vi "load.jsons.vi"() -> ()   [LabVIEW 2024]
uses:
  definitions/seriesJSON.ctl
  definitions/seriesInfo.ctl
  definitions/issueInfo.ctl
  definitions/creator.ctl
  definitions/character.ctl
  definitions/team.ctl
  definitions/location.ctl
  definitions/concept.ctl
  definitions/thing.ctl
  definitions/storyArc.ctl
  <vilib>/addons/_JKI.lib/Serialization/JSON/JKI JSON Serialization.lvlib
  series_class/series_class.lvclass
panel:
  out "error out":errorcluster
  out "event map out":map{string, set{string}}(c390)
  out "current series":string
  out "char map out":map{string, set{string}}(c390)
  in  "Path":path=path "D:/Comics/data/comicvine"
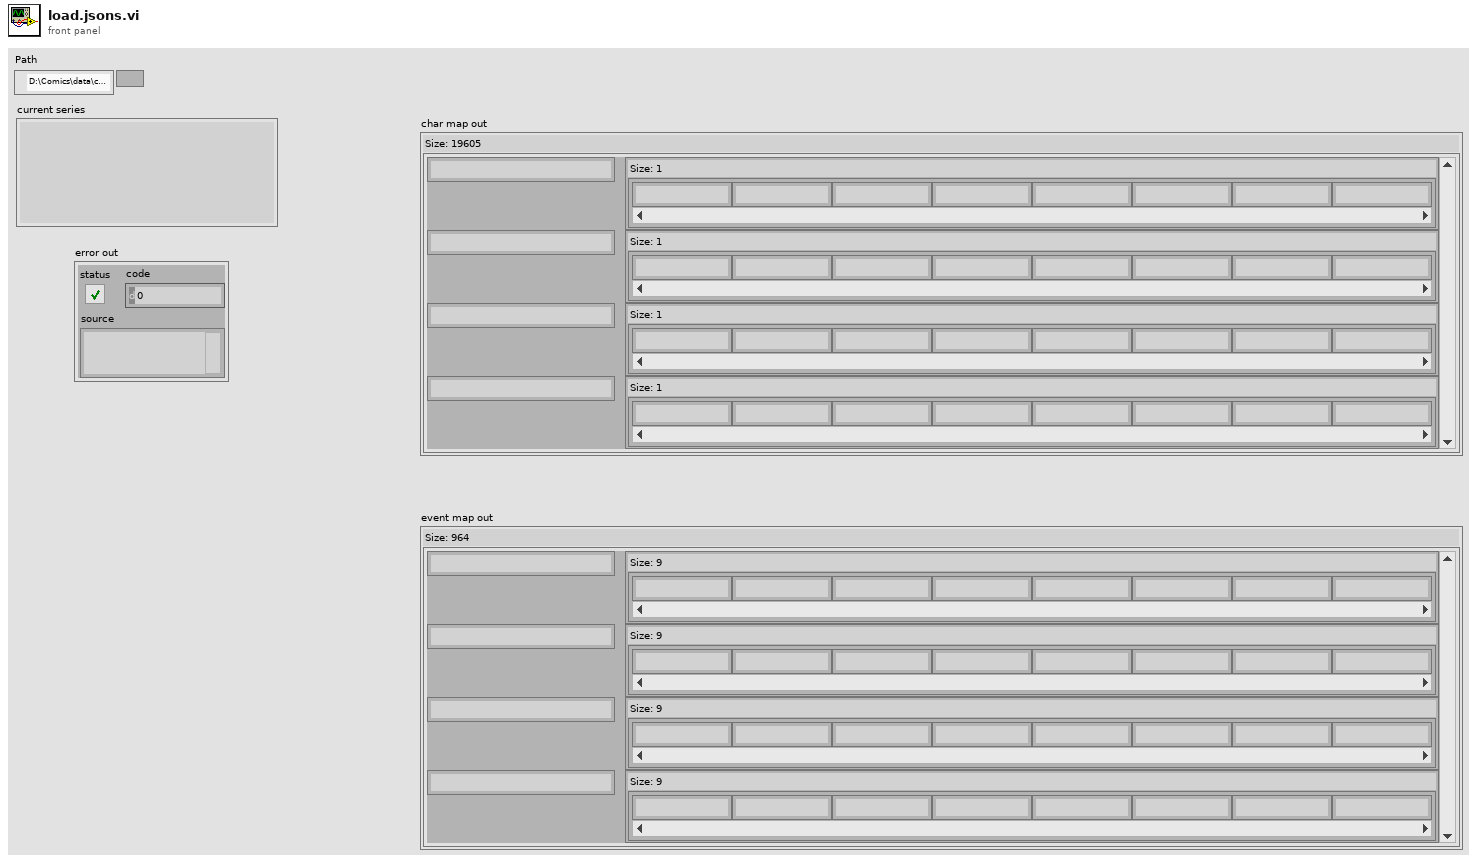
[diagram p1: front panel]
types:
  T1 = enum16{"open", "replace", "create", "open or create", "replace or create", "replace or create with confirmation"}
  T2 = cluster{"characters":cluster{"character":string, "issueIDs":string[]}[], "storyArcs":cluster{"storyArc":string, "issueIDs":string[]}[]}
  T3 = typedef "seriesJSON.ctl" = cluster{"seriesInfo":T4, "issueInfo":T5[]}
  T4 = typedef "seriesInfo.ctl" = cluster{"title":string, "base url":string, "publisher":string, "publisher url":string, "count":i32, "start year":i32, "volume":i32}
  T5 = typedef "issueInfo.ctl" = cluster{"cover date":timestamp, "release date":timestamp, "number":string, "url":string, "small cover url":string, "name":string, "large cover url":string, "id":string, "creators":T6[], "characters":T7[], "teams":T8[], "locations":T9[], "concepts":T10[], "objects":T11[], "storyArcs":T12[], "description":string}
  T6 = typedef "creator.ctl" = cluster{"name":string, "role":string, "url":string}
  T7 = typedef "character.ctl" = cluster{"name":string, "url":string}
  T8 = typedef "team.ctl" = cluster{"name":string, "url":string}
  T9 = typedef "location.ctl" = cluster{"name":string, "url":string}
  T10 = typedef "concept.ctl" = cluster{"name":string, "url":string}
  T11 = typedef "thing.ctl" = cluster{"name":string, "url":string}
  T12 = typedef "storyArc.ctl" = cluster{"name":string, "url":string}
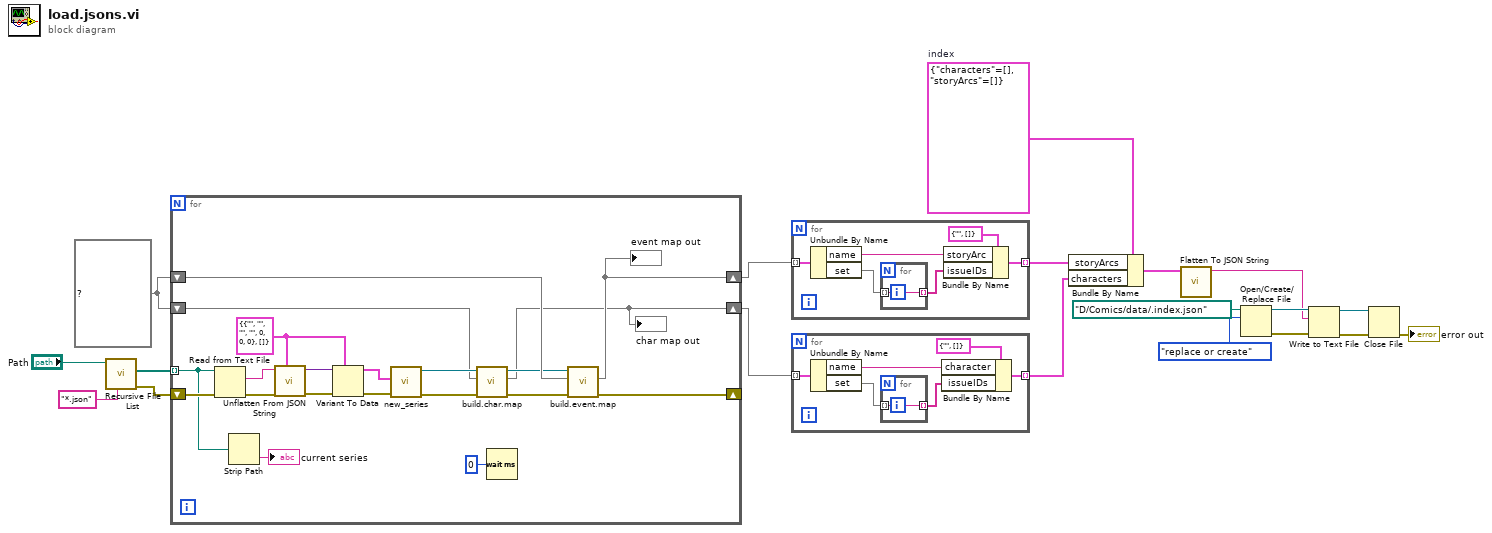
[diagram p0: block diagram]
diagram:
  w12 = T2 {"characters"=[], "storyArcs"=[]}  # index
  w15 = map{string, set{string}} {} ("char map in")
  n1 = call <vilib>:"Recursive File List.vi"("pattern"="*.json", "Folder Path"="Path") -> ("error out"=w16:errorcluster, "All Files in Dir"=w17:path[])  [unwired: 5 in, 3 out]
  n2 = for {
    tunnel: w17 -> [w28] mode=indexing
    shift-right: [w24] -> _
    shift-left: w16 -> [w39]
    shift-right: [w20] -> w13
    shift-left: w15 -> [w29]
    shift-right: [w21] -> w14
    shift-left: w15 -> [w23]
    w34 = T3 {"seriesInfo"={"title"="", "base url"="", "publisher"="", "publisher url"="", "count"=0, "start year"=0, "volume"=0}, "issueInfo"=[]} ("output cluster")
    n3 = Read from Text File(file (use dialog)=w28, error in=w39) -> (text=w38:string, error out=w37:errorcluster)  [unwired: 2 in, 2 out]
    n4 = Strip Path(path=w28) -> (name=→"current series":string)  [unwired: 1 out]
    n5 = call <vilib>:"Unflatten From JSON String.vi"("Type and Defaults"=w34, "error in (no error)"=w37, "JSON String"=w38) -> ("error out"=w36:errorcluster, "Variant"=w35:variant)  [unwired: 7 in]
    n6 = Variant To Data(error in=w36, type=w34, Variant=w35) -> (data=w32:T3, error out=w33:errorcluster)
    n7 = call "new_series.vi"("error in (no error)"=w33, "output cluster"=w32) -> ("error out"=w30:errorcluster, "series_class out"=w31:refnum<class "series_class.lvclass">)  [unwired: 8 in]
    n8 = call "build.char.map"("error in (no error)"=w30, "char map in"=w29, "series_class in"=w31) -> ("error out"=w25:errorcluster, "char map out"=w20:map{string, set{string}}, "series_class out"=w22:refnum<class "series_class.lvclass">)  [unwired: 6 in]
    "char map out" <- w20
    n9 = Wait (ms)(milliseconds to wait=u32 0) -> ()  [unwired: 1 out]
    n10 = call "build.event.map.vi"("error in (no error)"=w25, "event map in"=w23, "series_class in"=w22) -> ("error out"=w24:errorcluster, "event map out"=w21:map{string, set{string}})  [unwired: 6 in, 1 out]
    "event map out" <- w21
  }
  n11 = for {
    tunnel: w14 -> [w45] mode=indexing
    tunnel: [w40] -> w10 mode=indexing
    n12 = Unbundle By Name(w45) -> ("name"=w42:string, "set"=w44:set{string})
    n13 = for {
      tunnel: w44 -> [w46] mode=indexing
      tunnel: [w46] -> w41 mode=indexing
    }
    n14 = Bundle By Name(cluster=cluster{"storyArc":string, "issueIDs":string[]} {"storyArc"="", "issueIDs"=[]}, "storyArc"=w42, "issueIDs"=w41) -> (w40:cluster{"storyArc":string, "issueIDs":string[]})
  }
  n15 = for {
    tunnel: w13 -> [w52] mode=indexing
    tunnel: [w48] -> w11 mode=indexing
    n16 = Unbundle By Name(w52) -> ("name"=w50:string, "set"=w51:set{string})
    n17 = for {
      tunnel: w51 -> [w53] mode=indexing
      tunnel: [w53] -> w49 mode=indexing
    }
    n18 = Bundle By Name(cluster=cluster{"character":string, "issueIDs":string[]} {"character"="", "issueIDs"=[]}, "character"=w50, "issueIDs"=w49) -> (w48:cluster{"character":string, "issueIDs":string[]})
  }
  n19 = Bundle By Name(cluster=w12, "storyArcs"=w10, "characters"=w11) -> (w9:T2)
  n20 = call <vilib>:"Flatten To JSON String.vi"("Variant"=w9) -> ("JSON String"=w4:string)  [unwired: 9 in, 1 out]
  n21 = Open/Create/Replace File(file path (use dialog)=path "D:/Comics/data/.index.json", operation (0:open)=T1."replace or create") -> (refnum out=w5:refnum<file>, error out=w6:errorcluster)  [unwired: 4 in, 1 out]
  n22 = Write to Text File(file (use dialog)=w5, text=w4, error in=w6) -> (refnum out=w3:refnum<file>, error out=w2:errorcluster)  [unwired: 1 in, 1 out]
  n23 = Close File(refnum=w3, error in=w2) -> (error out=→"error out":errorcluster)  [unwired: 1 out]
